vi "getInitTime.vi"(8 "error in (no error)":errorcluster, 11 "Model in":refnum<class "Model.lvclass">) -> (0 "error out":errorcluster, 2 "initial Time":dbl, 3 "Model out":refnum<class "Model.lvclass">)   [LabVIEW 2016, in "Model.lvclass"]
uses:
  Model.lvclass
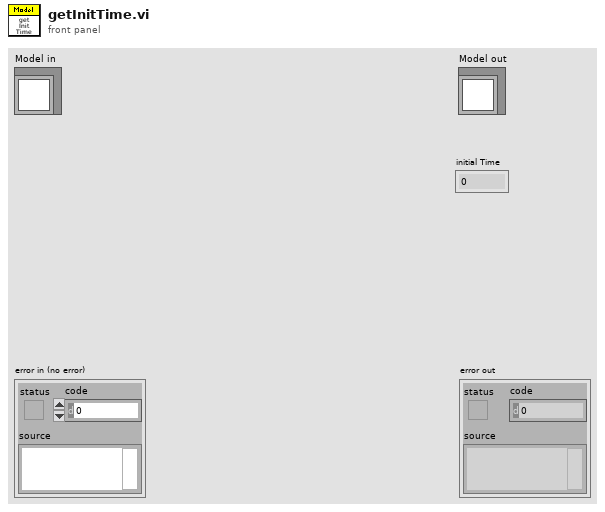
[diagram p1: front panel]
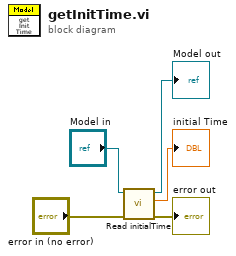
[diagram p0: block diagram]
diagram:
  n1 = call-dynamic "Read initialTime.vi"("error in (no error)"="error in (no error)", "Model in"="Model in") -> ("error out"=→"error out":errorcluster, "initial Time"=→"initial Time":dbl, "Model out"=→"Model out":refnum<class "Model.lvclass">)  [unwired: 7 in]
